vi "PTestbed_Cycling.vi"() -> ()   [LabVIEW 2020]
panel:
  out "DAQ error out":errorcluster[](array[cluster])
  out "PS error out":errorcluster[](array[cluster])
  in  "Battery Select":T1(ring)
  in  "Current Cutoff":dbl
  in  "Number of Cycles":i32
  in  "Charge filepath":path
  in  "Discharge filepath":path
  in  "Testname":string
  in  "Starting Cycle":i32
  out "PS Visa Out":refnum<visa-resource-name>
  out "parallel task out":refnum<k21>
  in  "Wait time":dbl
  in  "Discharge Current Setpoint":dbl format="%#.6g"
  in  "Charge Current Setpoint":dbl format="%#.6g"
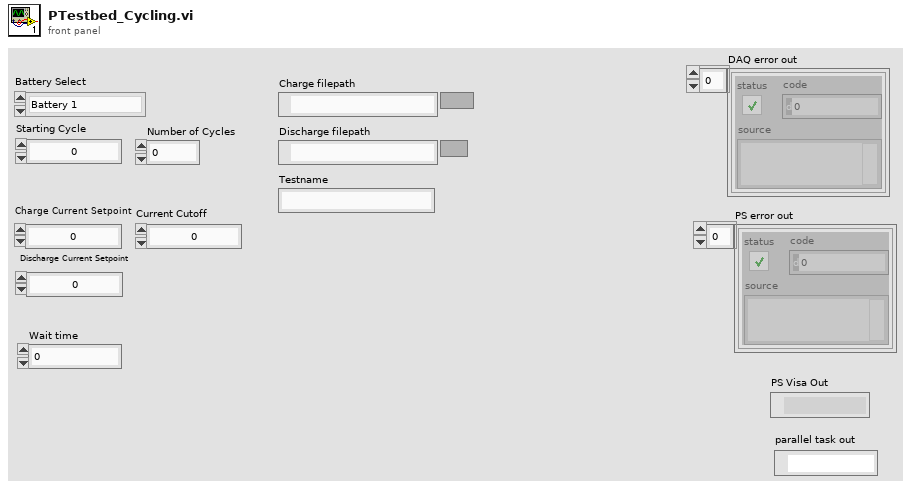
[diagram p1: front panel]
types:
  T1 = enum16{"Battery 1", "Battery 2", "Battery 3", "Battery 1&2", "Battery 1&3", "Battery 2&3", "Battery 1&2&3"}
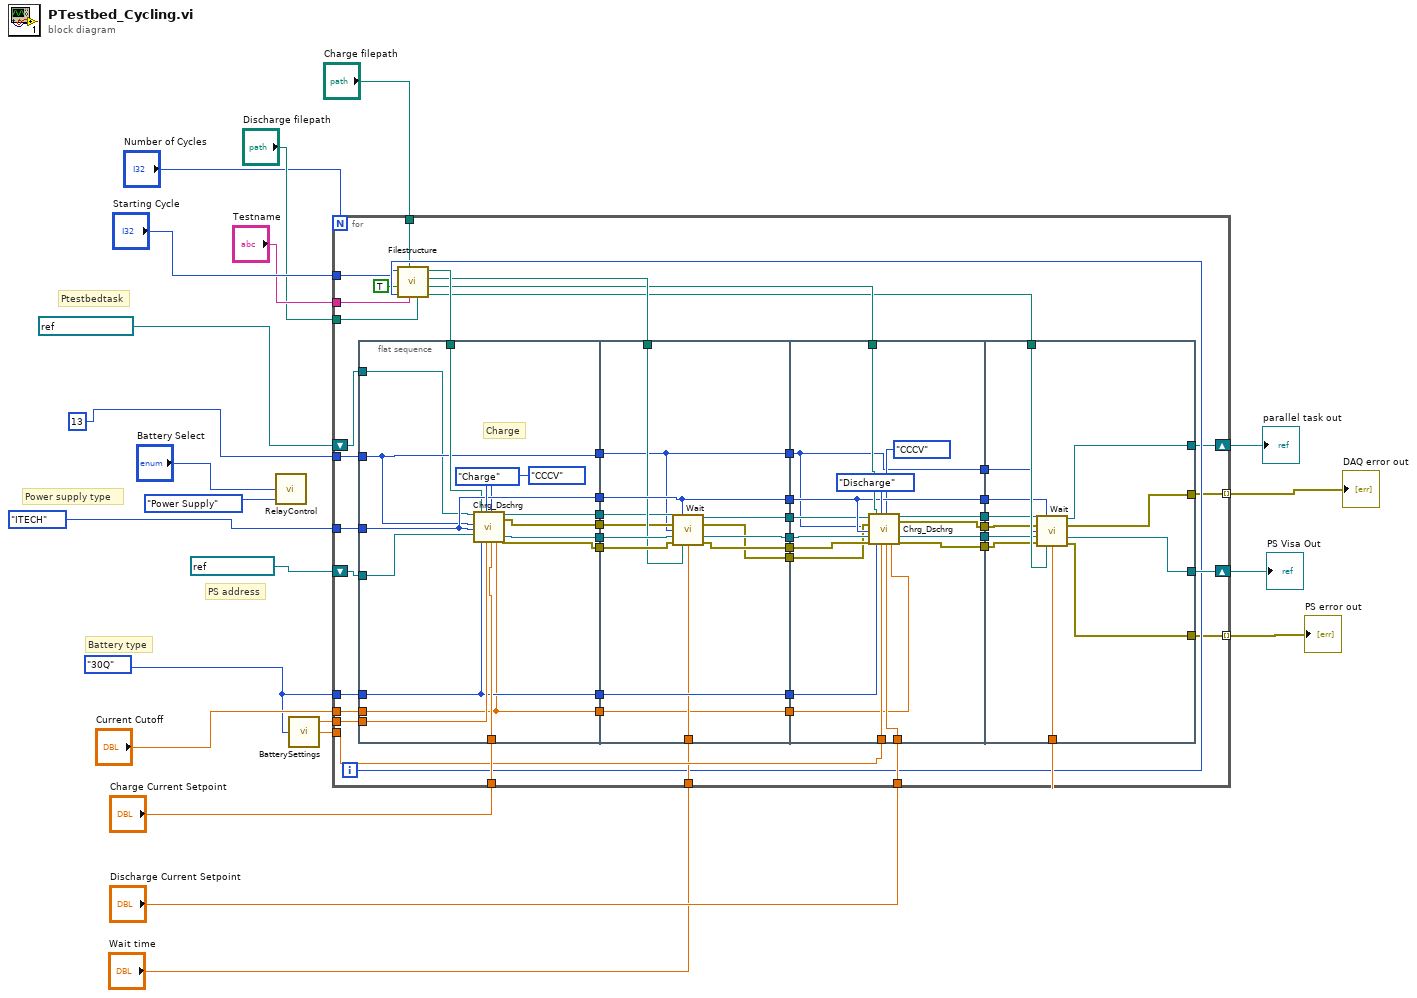
[diagram p0: block diagram]
diagram:
  w8 = enum16{"30Q", "40T"}."30Q" ("Battery Type")
  # "Battery type"
  # "PS address"
  # "Power supply type"
  # "Ptestbedtask"
  n1 = call "RelayControl.vi"("NHR or Battery Analyzer"=enum16{"Battery Analyzer", "Power Supply"}."Power Supply", "Battery Select"="Battery Select") -> ()  [unwired: 3 in]
  n2 = call "BatterySettings.vi"("Battery Type"=w8) -> ("Min Voltage (V)"=w20:dbl, "Max Voltage (V)"=w22:dbl)  [unwired: 2 in, 1 out]
  n3 = for {
    N: "Number of Cycles" -> [_]
    tunnel: 13 ("#DAQ outputs (1-13)") -> [w55]
    tunnel: enum16{"NHR", "ITECH"}."ITECH" ("PS type") -> [w54]
    tunnel: w22 -> [w52]
    tunnel: w8 -> [w51]
    tunnel: "Charge Current Setpoint" -> [w50]
    tunnel: w20 -> [w49]
    tunnel: "Discharge Current Setpoint" -> [w48]
    tunnel: "Wait time" -> [w43]
    shift-right: [w26] -> w16
    shift-left: refnum<k21> "PTesbedTask" ("Data Task in") -> [w56]
    shift-right: [w42] -> w17
    shift-left: refnum<visa-resource-name> "ITECH-PS3" ("PS Visa Out") -> [w53]
    tunnel: "Starting Cycle" -> [w40]
    tunnel: "Testname" -> [w38]
    tunnel: "Discharge filepath" -> [w37]
    tunnel: "Charge filepath" -> [w36]
    tunnel: "Current Cutoff" -> [w35]
    tunnel: [w24] -> w2 mode=indexing
    tunnel: [w23] -> w1 mode=indexing
    i -> [w41]
    n4 = flat-sequence {
      tunnel: w56 -> [w74]
      tunnel: w55 -> [w75]
      tunnel: w54 -> [w78]
      tunnel: w53 -> [w84]
      tunnel: w51 -> [w77]
      tunnel: w52 -> [w82]
      tunnel: w50 -> [w81]
      tunnel: [w80] -> w69
      tunnel: [w79] -> w68
      tunnel: [w78] -> w67
      tunnel: [w75] -> w66
      tunnel: [w77] -> w65
      tunnel: w47 -> [w76]
      tunnel: w35 -> [w72]
      tunnel: [w72] -> w34
      tunnel: [w71] -> w32
      tunnel: [w70] -> w31
      tunnel: w69 -> [w98]
      tunnel: w68 -> [w97]
      tunnel: w67 -> [w94]
      tunnel: [w96] -> w64
      tunnel: [w95] -> w63
      tunnel: w66 -> [w85]
      tunnel: [w85] -> w62
      tunnel: [w94] -> w61
      tunnel: w65 -> [w93]
      tunnel: [w93] -> w60
      tunnel: w46 -> [w92]
      tunnel: w43 -> [w91]
      tunnel: w34 -> [w90]
      tunnel: [w90] -> w33
      tunnel: w32 -> [w89]
      tunnel: w31 -> [w88]
      tunnel: [w87] -> w30
      tunnel: [w86] -> w29
      tunnel: w64 -> [w115]
      tunnel: w63 -> [w114]
      tunnel: w62 -> [w99]
      tunnel: w61 -> [w106]
      tunnel: w60 -> [w113]
      tunnel: w49 -> [w112]
      tunnel: w48 -> [w111]
      tunnel: w45 -> [w109]
      tunnel: [w108] -> w59
      tunnel: [w107] -> w58
      tunnel: [w106] -> w57
      tunnel: w33 -> [w104]
      tunnel: w30 -> [w103]
      tunnel: w29 -> [w102]
      tunnel: [w101] -> w28
      tunnel: [w100] -> w27
      tunnel: [w99] -> w25
      tunnel: w44 -> [w127]
      tunnel: w59 -> [w126]
      tunnel: w58 -> [w125]
      tunnel: w43 -> [w124]
      tunnel: w57 -> [w123]
      tunnel: [w122] -> w24
      tunnel: [w121] -> w42
      tunnel: w28 -> [w120]
      tunnel: w27 -> [w119]
      tunnel: [w118] -> w26
      tunnel: [w117] -> w23
      tunnel: w25 -> [w116]
      frame #0 {
        # "Charge"
        n5 = call "Chrg_Dschrg.vi"("Data Task in"=w74, "#DAQ outputs (1-13)"=w75, "PS type"=w78, "PS VISA in"=w84, "DischargeCyclePath"=w76, "Battery Type"=w77, "Charge/discharge"=enum8{"Charge", "Discharge"}."Charge", "Charge/Discharge Voltage Setpoint"=w82, "CC or CCCV"=enum16{"CC", "CCCV"}."CCCV", "Current Setpoint"=w81, "Current Cutoff"=w72) -> ("data task out"=w71:refnum<k21>, "data task error out"=w70:errorcluster, "PS VIS resource name out"=w80:refnum<visa-resource-name>, "PS error out"=w79:errorcluster)  [unwired: 5 in]
      }
      frame #1 {
        n6 = call "Wait.vi"("Data Task in"=w89, "PS type"=w94, "data task error in"=w88, "#DAQ outputs (1-13)"=w85, "PS VISA in"=w98, "PS error in"=w97, "Wait Filepath"=w92, "Wait time"=w91) -> ("data task out"=w87:refnum<k21>, "data task error out"=w86:errorcluster, "PS Visa Out"=w96:refnum<visa-resource-name>, "PS error out"=w95:errorcluster)  [unwired: 4 in]
      }
      frame #2 {
        n7 = call "Chrg_Dschrg.vi"("Data Task in"=w103, "data task error in"=w102, "#DAQ outputs (1-13)"=w99, "PS type"=w106, "PS VISA in"=w115, "PS error in"=w114, "DischargeCyclePath"=w109, "Battery Type"=w113, "Charge/discharge"=enum8{"Charge", "Discharge"}."Discharge", "Charge/Discharge Voltage Setpoint"=w112, "CC or CCCV"=enum16{"CC", "CCCV"}."CCCV", "Current Setpoint"=w111, "Current Cutoff"=w104) -> ("data task out"=w101:refnum<k21>, "data task error out"=w100:errorcluster, "PS VIS resource name out"=w108:refnum<visa-resource-name>, "PS error out"=w107:errorcluster)  [unwired: 3 in]
      }
      frame #3 {
        n8 = call "Wait.vi"("Data Task in"=w120, "PS type"=w123, "data task error in"=w119, "#DAQ outputs (1-13)"=w116, "PS VISA in"=w126, "PS error in"=w125, "Wait Filepath"=w127, "Wait time"=w124) -> ("data task out"=w118:refnum<k21>, "data task error out"=w117:errorcluster, "PS Visa Out"=w121:refnum<visa-resource-name>, "PS error out"=w122:errorcluster)  [unwired: 4 in]
      }
    }
    n9 = call "Filestructure.vi"("Discharge filepath"=w37, "Batteryname"=w38, "Charge filepath"=w36, "For loop i"=w41, "In for loop"=TRUE, "Starting Cycle"=w40) -> ("DischargeWaitPath"=w44:path, "DischargeCyclePath"=w45:path, "ChargeWaitPath"=w46:path, "ChargeCyclePath"=w47:path)  [unwired: 1 in, 1 out]
  }
  "PS Visa Out" <- w17
  "parallel task out" <- w16
  "PS error out" <- w2
  "DAQ error out" <- w1
